vi "Compare Multi-string Limit.vi"(2 "multi substring limit":string, 3 "result":string="ghj") -> (0 "limit":string="ghj", 1 "pass":bool)   [LabVIEW 2010]
doc: "This function searches for a key in a ..."
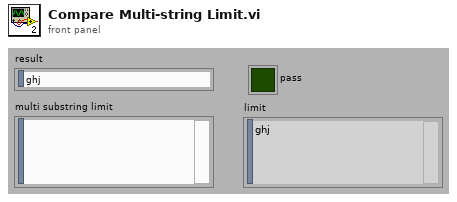
[diagram p1: front panel]
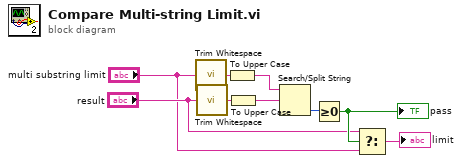
[diagram p0: block diagram]
diagram:
  n1 = call <vilib>:"Trim Whitespace.vi"("string"="multi substring limit") -> ("trimmed string"=w6:string)  [unwired: 1 in]
  n2 = call <vilib>:"Trim Whitespace.vi"("string"="result") -> ("trimmed string"=w8:string)  [unwired: 1 in]
  n3 = To Upper Case(1:w6) -> (0:w5:string)
  n4 = To Upper Case(1:w8) -> (0:w7:string)
  n5 = Search/Split String(string=w5, search string/char (-)=w7) -> (offset of match=w9:i32)  [unwired: 1 in, 2 out]
  n6 = Greater Or Equal To 0?(x=w9) -> (x >= 0?=w4:bool)
  "pass" <- w4
  n7 = Select(t="result", s=w4, f="multi substring limit") -> (s? t:f=→"limit":string)
